vi "Write Channel names.vi"(8 "error in (no error)":errorcluster, 10 "Channel names":string[](array[string]), 11 "DAQmx Digitizer in":refnum<class "DAQmx Digitizer.lvclass">) -> (0 "error out":errorcluster, 3 "DAQmx Digitizer out":refnum<class "DAQmx Digitizer.lvclass">)   [LabVIEW 2015]
uses:
  DAQmx Digitizer.lvclass
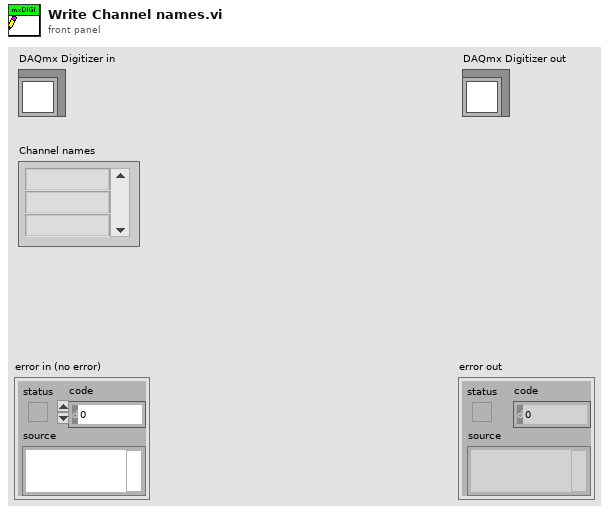
[diagram p1: front panel]
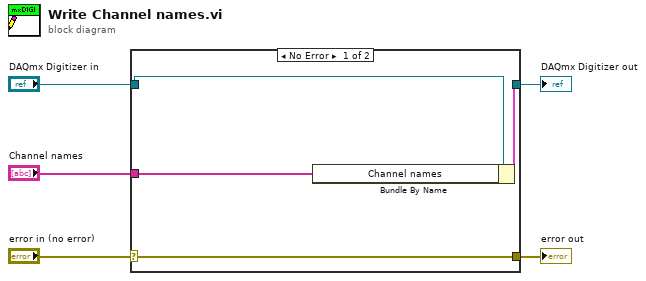
[diagram p0: block diagram]
diagram:
  n1 = case shown="No Error" "error in (no error)" {
    selector: "error in (no error)" -> [w9 w10]
    tunnel: [w9 w10] -> w4
    tunnel: [w7 w11] -> w2
    tunnel: "DAQmx Digitizer in" -> [w8 w11]
    tunnel: "Channel names" -> [w6 _]
    frame No Error {
      n2 = Bundle By Name(cluster=w8, "Channel names"=w6) -> (w7:cluster{})
    }
    frame Error {
    }
  }
  "error out" <- w4
  "DAQmx Digitizer out" <- w2
